vi "CMI ADS127L21 - Config Reference Clock Source.vi"(8 "error in (no error)":errorcluster, 9 "External Refclk Freq [Hz]":dbl=10000000.0, 10 "Use External Source? (False: Internal)":bool, 11 "session in":T1 {"channels"."Channel" min=1 max=8 step=1}) -> (0 "error out":errorcluster, 3 "session out":T1 {"channels"."Channel" min=1 max=8 step=1})   [LabVIEW 2020]
doc: "Select reference clock source."
uses:
  CMI ADS127L21 - Session.ctl
  CMI ADS127L21 - Record Channel.ctl
  CMI ADS127L21 - Input Range.ctl
  CMI ADS127L21 - Input Mode.ctl
  CMI ADS127L21 - Input Impedance.ctl
  CMI ADS127L21 - EXTOUT Mode.ctl
  CMI ADS127L21 - EXTOUT Polarity.ctl
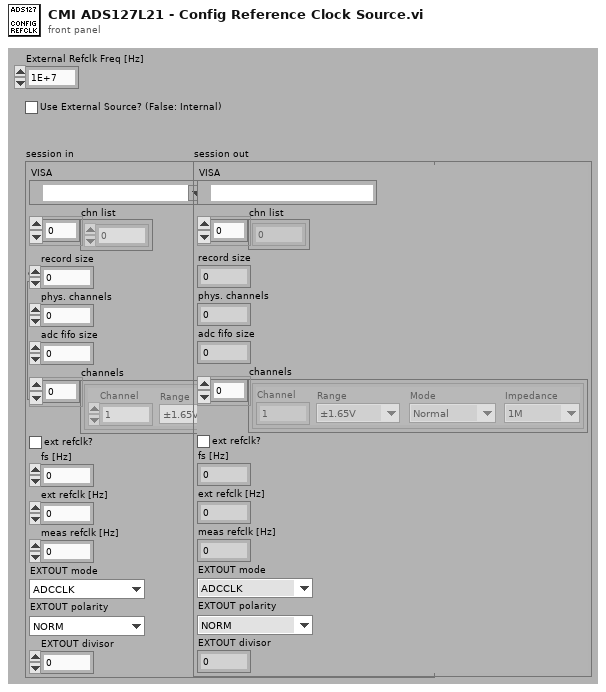
[diagram p1: front panel]
types:
  T1 = typedef "CMI ADS127L21 - Session.ctl" = cluster{"VISA":refnum<visa-resource-name>, "chn list":i32[], "record size":i32, "phys. channels":i32, "adc fifo size":i32, "channels":T2[], "ext refclk?":bool, "fs [Hz]":dbl, "ext refclk [Hz]":dbl, "meas refclk [Hz]":dbl, "EXTOUT mode":T6, "EXTOUT polarity":T7, "EXTOUT divisor":i32}
  T2 = typedef "CMI ADS127L21 - Record Channel.ctl" = cluster{"Range":T3, "Channel":i32, "Mode":T4, "Impedance":T5}
  T3 = typedef "CMI ADS127L21 - Input Range.ctl" = enum16{"±1.65V", "±2V"}
  T4 = typedef "CMI ADS127L21 - Input Mode.ctl" = enum16{"Normal", "Inverted", "GND"}
  T5 = typedef "CMI ADS127L21 - Input Impedance.ctl" = enum16{"1M", "1k5"}
  T6 = typedef "CMI ADS127L21 - EXTOUT Mode.ctl" = enum16{"ADCCLK", "REFCLK", "SMPLCLK", "FIRST"}
  T7 = typedef "CMI ADS127L21 - EXTOUT Polarity.ctl" = enum16{"NORM", "INV"}
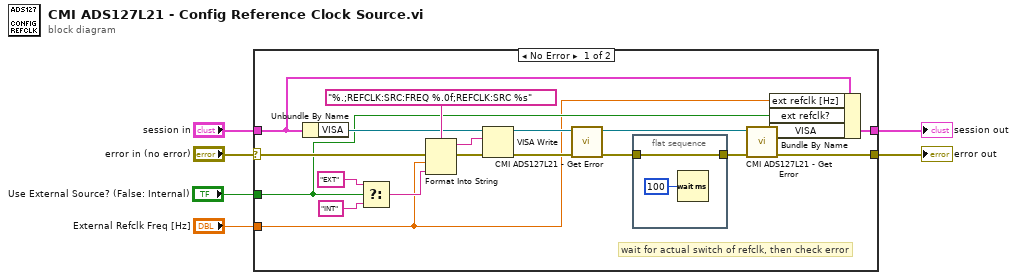
[diagram p0: block diagram]
diagram:
  n1 = case shown="No Error" "error in (no error)" {
    selector: "error in (no error)" -> [w20 w29]
    tunnel: "session in" -> [w17 w28]
    tunnel: [w18 w28] -> w5
    tunnel: [w12 w29] -> w4
    tunnel: "Use External Source? (False: Internal)" -> [w9 _]
    tunnel: "External Refclk Freq [Hz]" -> [w7 _]
    frame No Error {
      # "wait for actual switch of refclk, then check error"
      n2 = Unbundle By Name(w17) -> ("VISA"=w19:refnum<visa-resource-name>)
      n3 = Select(t="EXT", s=w9, f="INT") -> (s? t:f=w8:string)
      n4 = Format Into String(format string="%.;REFCLK:SRC:FREQ %.0f;REFCLK:SRC %s", error in=w20, w7, w8) -> (resulting string=w21:string, error out=w24:errorcluster)  [unwired: 1 in]
      n5 = VISA Write(VISA resource name=w19, write buffer=w21, error in (no error)=w24) -> (VISA resource name out=w22:refnum<visa-resource-name>, error out=w23:errorcluster)  [unwired: 1 out]
      n6 = call "CMI ADS127L21 - Get Error.vi"("error in (no error)"=w23, "VISA in"=w22) -> ("error out"=w14:errorcluster, "VISA out"=w10:refnum<visa-resource-name>)  [unwired: 8 in]
      n7 = flat-sequence {
        tunnel: w14 -> [w27]
        tunnel: [w27] -> w13
        frame #0 {
          n8 = Wait (ms)(milliseconds to wait=u32 100) -> ()  [unwired: 1 out]
        }
      }
      n9 = call "CMI ADS127L21 - Get Error.vi"("error in (no error)"=w13, "VISA in"=w10) -> ("error out"=w12:errorcluster, "VISA out"=w11:refnum<visa-resource-name>)  [unwired: 8 in]
      n10 = Bundle By Name(cluster=w17, "ext refclk [Hz]"=w7, "ext refclk?"=w9, "VISA"=w11) -> (w18:T1)
    }
    frame Error {
    }
  }
  "error out" <- w4
  "session out" <- w5
